vi "example_3_fg_execution.vi"() -> ()   [LabVIEW 2015, in "lv_mutex_shared_1.lvlib"]
uses:
  lv_mutex_shared_1.lvlib
panel:
  in  "Enable Parallel Instances?":bool
  out "Equal to Initial Value?":bool
  out "Initailized Value":dbl
  out "Data Read":dbl[](array[numeric])
  in  "FG Execution Mode":T1(radio)
  # "This VI shows how a VI that stores data will act when there are multiple\ninstances when different execution modes are selected: Configure the\nVI and run:\n*Configure execution mode to run instances of the functional global\n as configured.\n*Update the number of times to execute to run multiple iterations\n*Enable parallel instances to choose how the for loop is configured."
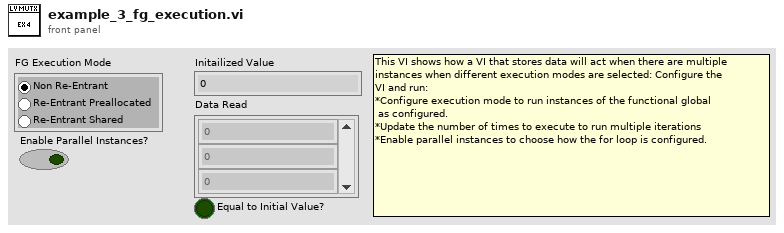
[diagram p1: front panel]
types:
  T1 = enum32{"Non Re-Entrant", "Re-Entrant Preallocated", "Re-Entrant Shared"}
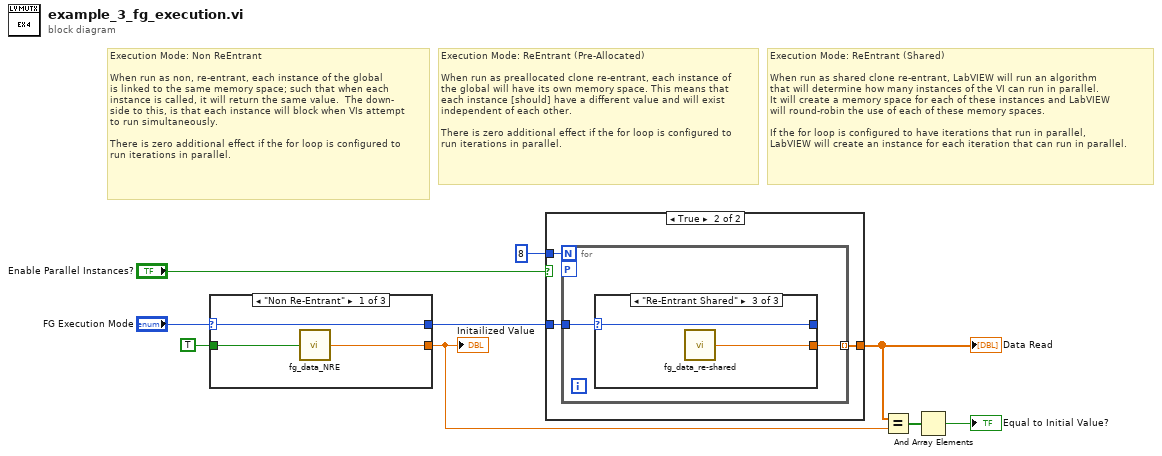
[diagram p0: block diagram]
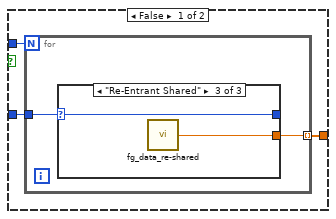
[diagram p2: hidden frame]
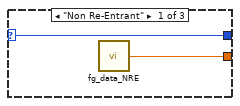
[diagram p3: hidden frame]
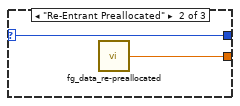
[diagram p4: hidden frame]
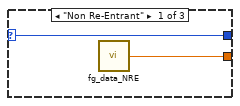
[diagram p5: hidden frame]
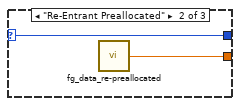
[diagram p6: hidden frame]
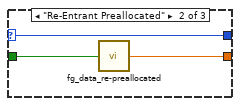
[diagram p7: hidden frame]
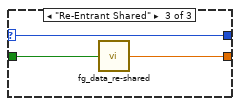
[diagram p8: hidden frame]
diagram:
  # "Execution Mode: ReEntrant (Shared)\n\nWhen run as shared clone re-entrant, LabVIEW will run an algorithm\nthat will determine how many instances of the VI can run in parallel.\nIt will create a memory space for each of these instances and LabVIEW\nwill round-robin the use of each of these memory spaces. \n\nIf the for loop is configured to have iterations that run in parallel,\nLabVIEW will create an instance for each iteration that can run in parallel."
  # "Execution Mode: ReEntrant (Pre-Allocated)\n\nWhen run as preallocated clone re-entrant, each instance of\nthe global will have its own memory space. This means that\neach instance [should] have a different value and will exist\nindependent of each other.\n\nThere is zero additional effect if the for loop is configured to\nrun iterations in parallel."
  # "Execution Mode: Non ReEntrant\n\nWhen run as non, re-entrant, each instance of the global\nis linked to the same memory space; such that when each\ninstance is called, it will return the same value.  The down-\nside to this, is that each instance will block when VIs attempt\nto run simultaneously.\n\nThere is zero additional effect if the for loop is configured to\nrun iterations in parallel."
  n1 = case shown="\"Non Re-Entrant\"" "FG Execution Mode" {
    selector: "FG Execution Mode" -> [w12 w15 w18]
    tunnel: [w12 w15 w18] -> w7
    tunnel: TRUE -> [w11 w14 w17]
    tunnel: [w10 w13 w16] -> w4
    frame "Non Re-Entrant" {
      n2 = call "fg_data_NRE.vi"("initialize?"=w11) -> ("data out"=w10:dbl)
    }
    frame "Re-Entrant Preallocated" {
      n3 = call "fg_data_re-preallocated.vi"("initialize?"=w14) -> ("data out"=w13:dbl)
    }
    frame "Re-Entrant Shared" {
      n4 = call "fg_data_re-shared.vi"("initialize?"=w17) -> ("data out"=w16:dbl)
    }
  }
  "Initailized Value" <- w4
  n5 = case shown="True" "Enable Parallel Instances?" {
    tunnel: 8 ("# of Times to Execute") -> [w21 w32]
    tunnel: w7 -> [w20 w31]
    tunnel: [w19 w30] -> w5
    frame False {
      n6 = for {
        N: w21 -> [_]
        tunnel: w20 -> [w23]
        tunnel: [w22] -> w19 mode=indexing
        n7 = case shown="\"Re-Entrant Shared\"" w23 {
          selector: w23 -> [w25 w27 w29]
          tunnel: [w25 w27 w29] -> _
          tunnel: [w24 w26 w28] -> w22
          frame "Non Re-Entrant" {
            n8 = call "fg_data_NRE.vi"() -> ("data out"=w24:dbl)  [unwired: 1 in]
          }
          frame "Re-Entrant Preallocated" {
            n9 = call "fg_data_re-preallocated.vi"() -> ("data out"=w26:dbl)  [unwired: 1 in]
          }
          frame "Re-Entrant Shared" {
            n10 = call "fg_data_re-shared.vi"() -> ("data out"=w28:dbl)  [unwired: 1 in]
          }
        }
      }
    }
    frame True {
      n11 = for {
        N: w32 -> [_]
        tunnel: w31 -> [w34]
        tunnel: [w33] -> w30 mode=indexing
        workers-P: _ -> [_]
        n12 = case shown="\"Re-Entrant Shared\"" w34 {
          selector: w34 -> [w36 w38 w40]
          tunnel: [w36 w38 w40] -> _
          tunnel: [w35 w37 w39] -> w33
          frame "Non Re-Entrant" {
            n13 = call "fg_data_NRE.vi"() -> ("data out"=w35:dbl)  [unwired: 1 in]
          }
          frame "Re-Entrant Preallocated" {
            n14 = call "fg_data_re-preallocated.vi"() -> ("data out"=w37:dbl)  [unwired: 1 in]
          }
          frame "Re-Entrant Shared" {
            n15 = call "fg_data_re-shared.vi"() -> ("data out"=w39:dbl)  [unwired: 1 in]
          }
        }
      }
    }
  }
  "Data Read" <- w5
  n16 = Equal?(x=w5, y=w4) -> (x = y?=w3:bool[])
  n17 = And Array Elements(Boolean array=w3) -> (logical AND=→"Equal to Initial Value?":bool)
